vi "Arm Transfer R to F.vi"() -> ()   [LabVIEW 2015]
uses:
  Typedef/IntakeControllerActions.ctl
  Typedef/IntakeControllerMsg.ctl
  ArmController/ArmController.lvlib
panel:
  in  "milliseconds to wait 2":u32=800
  in  "milliseconds to wait":u32=250
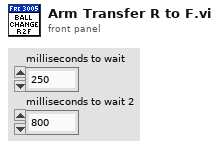
[diagram p1: front panel]
types:
  T1 = typedef "IntakeControllerMsg.ctl" = cluster{"Cmd":T2, "Data":variant}
  T2 = typedef "IntakeControllerActions.ctl" = enum16{"Wait on Intake Rear", "Wait on Angle Rear", "Go To Angle Rear", "Wait on Intake Front", "Wait on Angle Front", "Set Roller Front", "Set Roller Rear", "Go To Angle Front", "Wait ms"}
  T3 = cluster{"Down":dbl, "Pickup":dbl, "Shoot":dbl, "Turtle":dbl, "Intake Block":dbl, "Intake Transfer":dbl}
  T4 = cluster{"Down":dbl, "Pickup":dbl, "Shoot":dbl, "Turtle":dbl}
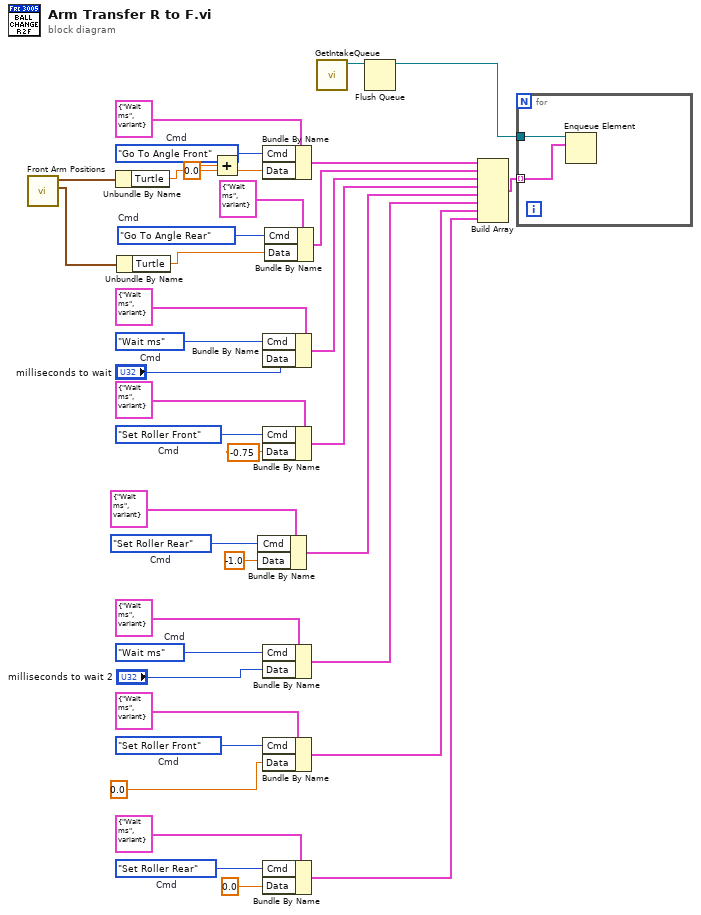
[diagram p0: block diagram]
diagram:
  w6 = IntakeControllerActions."Set Roller Rear"  # Cmd
  w13 = IntakeControllerActions."Go To Angle Rear"  # Cmd
  w39 = IntakeControllerActions."Set Roller Rear"  # Cmd
  w31 = IntakeControllerActions."Set Roller Front"  # Cmd
  w35 = IntakeControllerActions."Wait ms"  # Cmd
  w28 = IntakeControllerActions."Set Roller Front"  # Cmd
  w23 = IntakeControllerActions."Wait ms"  # Cmd
  w20 = IntakeControllerActions."Go To Angle Front"  # Cmd
  n1 = call "Front Arm Positions.vi"() -> ("Rear Arm"=w10:T3, "Front Arm"=w15:T4)  [unwired: 10 in]
  n2 = Unbundle By Name(w15) -> ("Turtle"=w16:dbl)
  n3 = Unbundle By Name(w10) -> ("Turtle"=w9:dbl)
  n4 = Add(x=0.0, y=w16) -> (x+y=w2:dbl)
  n5 = Bundle By Name(cluster=T1 {"Cmd"=enum."Wait ms", "Data"=variant(i32 50)} ("output cluster"), "Cmd"=w6, "Data"=-1.0) -> (w4:T1)
  n6 = Bundle By Name(cluster=T1 {"Cmd"=enum."Wait ms", "Data"=variant(i32 50)} ("output cluster"), "Cmd"=w20, "Data"=w2) -> (w22:T1)
  n7 = Bundle By Name(cluster=T1 {"Cmd"=enum."Wait ms", "Data"=variant(i32 50)} ("output cluster"), "Cmd"=w23, "Data"="milliseconds to wait") -> (w26:T1)
  n8 = Bundle By Name(cluster=T1 {"Cmd"=enum."Wait ms", "Data"=variant(i32 50)} ("output cluster"), "Cmd"=w28, "Data"=-0.75) -> (w29:T1)
  n9 = Bundle By Name(cluster=T1 {"Cmd"=enum."Wait ms", "Data"=variant(i32 50)} ("output cluster"), "Cmd"=w35, "Data"="milliseconds to wait 2") -> (w3:T1)
  n10 = Bundle By Name(cluster=T1 {"Cmd"=enum."Wait ms", "Data"=variant(i32 50)} ("output cluster"), "Cmd"=w31, "Data"=0.0 ("Diffs")) -> (w37:T1)
  n11 = Bundle By Name(cluster=T1 {"Cmd"=enum."Wait ms", "Data"=variant(i32 50)} ("output cluster"), "Cmd"=w39, "Data"=0.0 ("Diffs")) -> (w18:T1)
  n12 = Bundle By Name(cluster=T1 {"Cmd"=enum."Wait ms", "Data"=variant(i32 50)} ("output cluster"), "Cmd"=w13, "Data"=w9) -> (w11:T1)
  n13 = call "GetIntakeQueue.vi"() -> ("queue out"=w19:refnum<queue>)  [unwired: 11 in]
  n14 = Flush Queue(queue=w19) -> (queue out=w17:refnum<queue>)  [unwired: 1 in, 2 out]
  n15 = Build Array(w22, w11, w26, w29, w4, w3, w37, w18) -> (w30:T1[])
  n16 = for {
    tunnel: w17 -> [w41]
    tunnel: w30 -> [w40] mode=indexing
    n17 = Enqueue Element(queue=w41, element=w40) -> ()  [unwired: 2 in, 3 out]
  }
